vi "TAMANHO-CLIENTE 2.vi"() -> ()   [LabVIEW 2019]
panel:
  out "size":i32
  in  "stop":bool
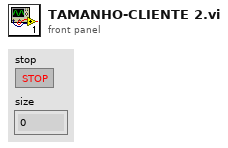
[diagram p1: front panel]
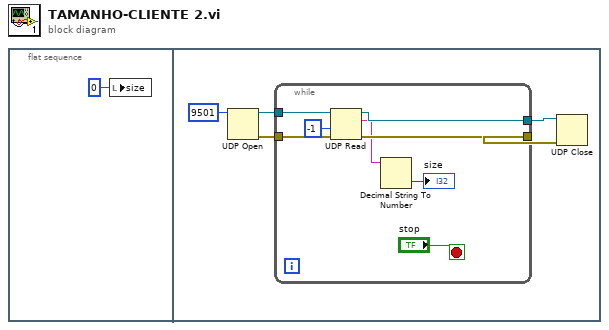
[diagram p0: block diagram]
diagram:
  n1 = flat-sequence {
    frame #0 {
      n2 = local write "size"(0 ("size")) -> ()
    }
    frame #1 {
      n3 = UDP Open(11:u16 9501 ("port")) -> (port=w6:refnum<k16>, 0:w5:errorcluster)  [unwired: 4 in, 1 out]
      n4 = while {
        tunnel: w6 -> [w13]
        tunnel: w5 -> [w12]
        tunnel: [w11] -> w4
        tunnel: [w10] -> w3
        stop <- "stop" stop-if-true
        n5 = UDP Read(connection ID=w13, timeout ms (25000)=-1, 8:w12) -> (data out=w8:string, error out=w10:errorcluster, 3:w11:refnum<k16>)  [unwired: 1 in, 2 out]
        n6 = Decimal String To Number(string=w8) -> (number=→"size":i32)  [unwired: 2 in, 1 out]
      }
      n7 = UDP Close(connection ID=w4, 8:w3) -> ()  [unwired: 2 out]
    }
  }
